vi "Set Setpoint.vi"(9 "value":variant, 10 "Point":string, 11 "Task Base in":refnum<class "Task Base.lvclass">) -> (3 "Task Base out":refnum<class "Task Base.lvclass">)   [LabVIEW 2023, in "Task Base.lvclass"]
uses:
  Task Base.lvclass
  Task Base.lvclass/Task Base.ctl
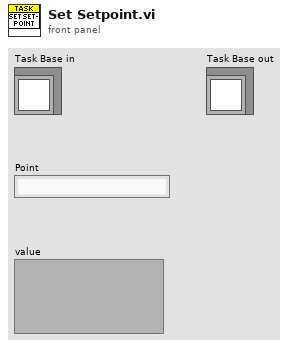
[diagram p1: front panel]
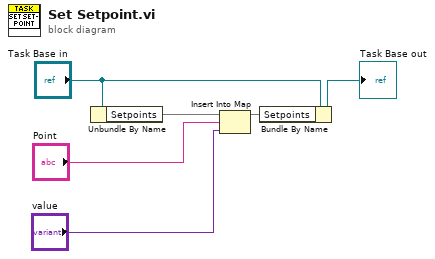
[diagram p0: block diagram]
diagram:
  n1 = Unbundle By Name("Task Base in") -> ("Setpoints"=w6:map{string, variant})
  n2 = Insert Into Map(map in=w6, key="Point", value="value") -> (map out=w3:map{string, variant})  [unwired: 2 out]
  n3 = Bundle By Name(cluster="Task Base in", "Setpoints"=w3) -> (→"Task Base out":refnum<class "Task Base.lvclass">)
